vi "Optics_CreateMessageQueues.vi"(8 "error in (no error)":errorcluster) -> (0 "error out":errorcluster, 3 "Message Queues out":T1)   [LabVIEW 2021]
doc: "This VI creates and initializes all the message queues for your application. If your application requires more than one message queue, right-click the \"Message Queues\" constant above and select Open Type Def. Add the new Message Queue(s) to the type definition, then initialize them in this VI."
uses:
  Controls/Optics_MessageQueues.ctl
  full-duck/Files/Support/Message Queue/Controls/Message Cluster.ctl
  full-duck/Files/Support/Message Queue/Message_queue_library.lvlib
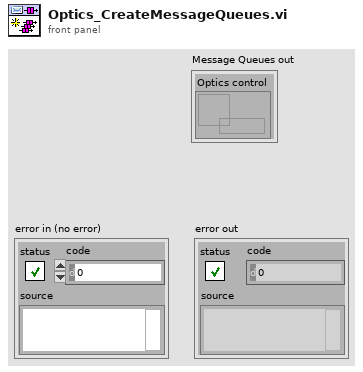
[diagram p1: front panel]
types:
  T1 = typedef "Optics_MessageQueues.ctl" = cluster{"Optics control":refnum<queue>}
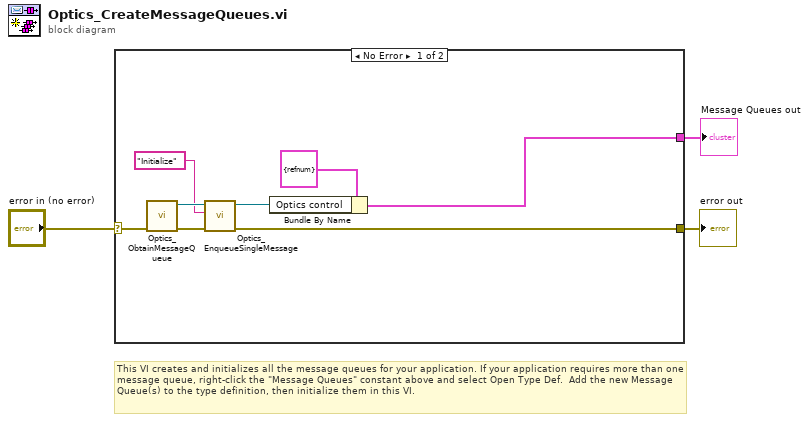
[diagram p0: block diagram]
diagram:
  # "This VI creates and initializes all the message queues for your application. If your application requires more than one message queue, right-click the \"Message Queues\" constant above and select Open Type Def.  Add the new Message Queue(s) to the type definition, then initialize them in this VI."
  n1 = case shown="No Error" "error in (no error)" {
    selector: "error in (no error)" -> [w8 w12]
    tunnel: [w7 w12] -> w2
    tunnel: [w5 _] -> w1
    frame No Error {
      n2 = call "Optics_ObtainMessageQueue.vi"("error in (no error)"=w8) -> ("error out"=w11:errorcluster, "Message Queue"=w10:refnum<queue>)  [unwired: 9 in]
      n3 = call "Optics_EnqueueSingleMessage.vi"("error in (no error)"=w11, "Message"="Initialize", "Message Queue"=w10) -> ("error out"=w7:errorcluster, "dup Message Queue"=w9:refnum<queue>)  [unwired: 7 in]
      n4 = Bundle By Name(cluster=T1 {"Optics control"=refnum} ("Message Queues"), "Optics control"=w9) -> (w5:T1)
    }
    frame Error {
    }
  }
  "error out" <- w2
  "Message Queues out" <- w1
